vi "OpenMovieFile.vi"(0 "Path":path) -> (1 "error out":errorcluster, 2 "# frames":dbl, 3 "QT Ref Out":T1)   [LabVIEW 2024]
doc: "This VI will initialize a sequence of vi’s for reading frames from a movie file."
uses:
  <userlib>/ImageProcessing/QTLIB_2595_LV86/QT_Private.ctl
  <userlib>/ImageProcessing/QTLIB_2595_LV86/QT_File.ctl
  <userlib>/ImageProcessing/QTLIB_2595_LV86/QT_FrameSelector.ctl
  <userlib>/ImageProcessing/QTLIB_2595_LV86/QT_Track.ctl
  <userlib>/ImageProcessing/QTLIB_2595_LV86/QT_MovieInfo.ctl
  <userlib>/ImageProcessing/QTLIB_2595_LV86/QT_Ref.ctl
panel:
  out "total time (s)":dbl
  out "Movie info":T2 {"Tracks"."Rate" format="%.2f"}
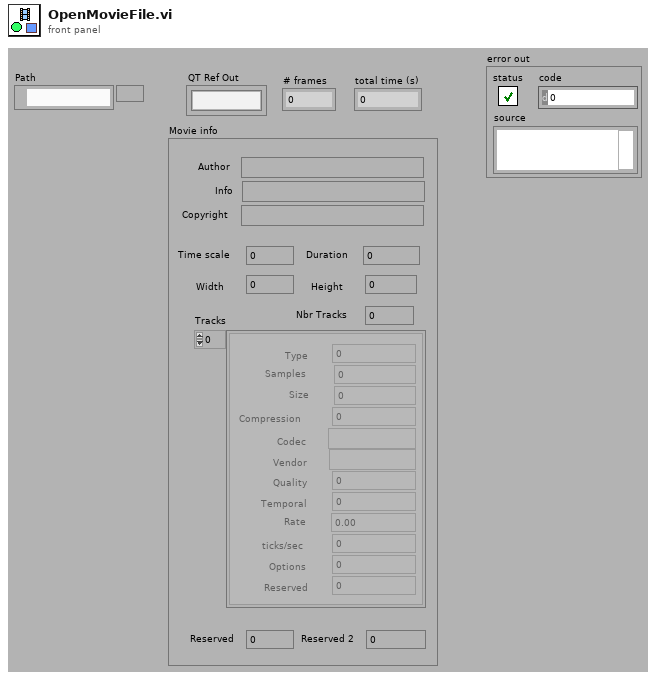
[diagram p1: front panel]
types:
  T1 = typedef "QT_Ref.ctl" = refnum<k1>
  T2 = typedef "QT_MovieInfo.ctl" = cluster{"Author":string, "Info":string, "Copyright":string, "Time scale":i32, "Duration":i32, "Width":i32, "Height":i32, "Nbr Tracks":i32, "Tracks":T3[], "Reserved":i32, "Reserved 2":i32}
  T3 = typedef "QT_Track.ctl" = cluster{"Type":i32, "Samples":i32, "Size":i32, "Compression":i32, "Codec":string, "Vendor":string, "Quality":i32, "Temporal":i32, "Rate ":dbl, "ticks/sec":i32, "Options":i32, "Reserved":i32}
  T4 = typedef "QT_FrameSelector.ctl" = enum32{"Get Next Frame", "Get Prev Frame", "Get Last Frame", "Get First Frame", "Get Frame ID", "Get Frame at Time", "reserved"}
  T5 = typedef "QT_File.ctl" = cluster{"Paths":string[], "Options":i32, "Dialogs":u32, "Reserved":i32}
  T6 = typedef "QT_Private.ctl" = cluster{"reserved 1":i32, "reserved 2":i32, "reserved 3":i32, "reserved 4":i32}
  T7 = typedef "QT_Image.ctl" = cluster{"Width":i32, "Height":i32, "Depth":i32, "data":u8[], "Compressed data":u8[], "Color table":u32[], "Duration":i32, "Options":i32, "Timestamp":i32, "ID":i32, "Reserved":i32, "Dialogs":u32}
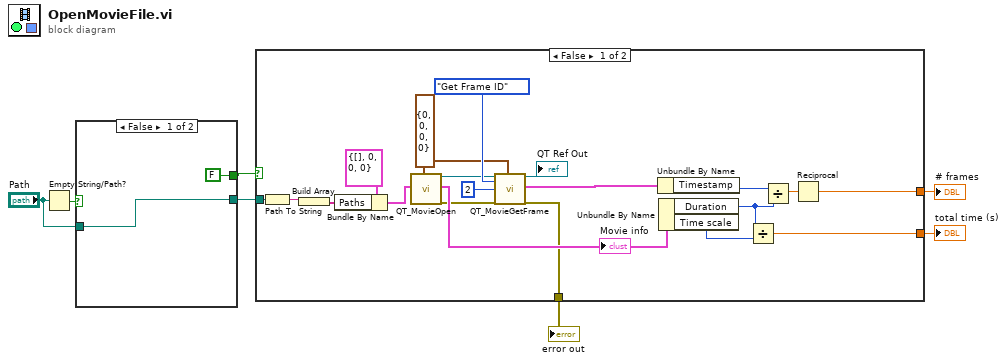
[diagram p0: block diagram]
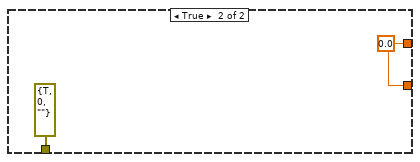
[diagram p2: hidden frame]
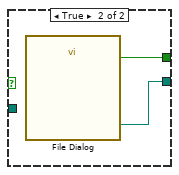
[diagram p3: hidden frame]
diagram:
  n1 = Empty String/Path?(string/path="Path") -> (empty?=w7:bool)
  n2 = case shown="False" w7 {
    tunnel: [FALSE ("cancelled") w11] -> w6
    tunnel: [w9 w10] -> w5
    tunnel: "Path" -> [w9 _]
    frame False {
    }
    frame True {
      n3 = call "File Dialog"() -> ("selected path"=w10:path, "cancelled"=w11:bool)  [unwired: 12 in, 2 out]
    }
  }
  n4 = case shown="False" w6 {
    tunnel: w5 -> [w15 _]
    tunnel: [w14 errorcluster {"status"=TRUE, "code"=0, "source"=""} ("error out")] -> w3
    tunnel: [w13 w33] -> w2
    tunnel: [w12 w33] -> w1
    frame False {
      w18 = T6 {"reserved 1"=0, "reserved 2"=0, "reserved 3"=0, "reserved 4"=0} ("Private")
      n5 = Path To String(path=w15) -> (string=w31:string)
      n6 = Build Array(w31) -> (w30:string[])
      n7 = Bundle By Name(cluster=T5 {"Paths"=[], "Options"=0, "Dialogs"=0, "Reserved"=0} ("File Settings"), "Paths"=w30) -> (w29:T5)
      n8 = call <userlib>:"QT_MovieOpen.vi"("File Settings"=w29, "Private"=w18) -> ("QT Ref Out"=w21:T1, "Movie info"=w26:T2, "error out"=w17:errorcluster)  [unwired: 15 in]
      "Movie info" <- w26
      n9 = call <userlib>:"QT_MovieGetFrame.vi"("QT Ref In"=w21, "Frame Access"=QT_FrameSelector."Get Frame ID", "Frame ID"=2, "error in"=w17, "Private"=w18) -> ("QT Ref Out"=→"QT Ref Out":T1, "Image Out"=w16:T7, "error out"=w14:errorcluster)  [unwired: 12 in]
      n10 = Unbundle By Name(w16) -> ("Timestamp"=w23:i32)
      n11 = Unbundle By Name(w26) -> ("Duration"=w20:i32, "Time scale"=w27:i32)
      n12 = Divide(x=w20, y=w27) -> (x/y=w12:dbl)
      n13 = Divide(x=w23, y=w20) -> (x/y=w22:dbl)
      n14 = Reciprocal(x=w22) -> (1/x=w13:dbl)
    }
    frame True {
      w33 = 0.0
    }
  }
  "error out" <- w3
  "# frames" <- w2
  "total time (s)" <- w1
